vi "Read Parameter from Word.vi"(8 "error in":errorcluster, 9 "parameter definition":T1={"start index"=10, "size"=19, "encoding"=enum."BNR", "signed"=FALSE, "scale multiplier"=1.0, "scale offset"=0.0}, 11 "32-bit Word in":refnum<class "32-bit Word.lvclass">) -> (0 "error out":errorcluster, 2 "parameter value":dbl, 3 "32-bit Word out":refnum<class "32-bit Word.lvclass">)   [LabVIEW 2020, in "32-bit Word.lvclass"]
uses:
  32-bit Word.lvclass
  Parameter Definition.ctl
  Encoding and Decoding/Encoding.ctl
  32-bit Word.lvclass/32-bit Word.ctl
  696e3cb6-aa1b-4579-a134-6b36b9c1fdc9.vi
  8302f7cf-3c99-45e8-838e-289f83284f96.vi
  Read 32-Bit Word.vi
  696e3cb6-aa1b-4579-a134-6b36b9c1fdc9.vi/16a2565b-3c16-407b-a626-9da2a3da432e.vi
  8302f7cf-3c99-45e8-838e-289f83284f96.vi/0a001d06-2809-4638-8d0b-e017d2157007.vi
  Encoding and Decoding/BCD Decode Integer.vi
  Encoding and Decoding/BCD Decode Integer.vi/9a65bfc0-0d77-4ef3-ab58-63df1e1caa90.vi
  ARINC 429.lvclass
  Encoding and Decoding/Encoding and Decoding.lvlib
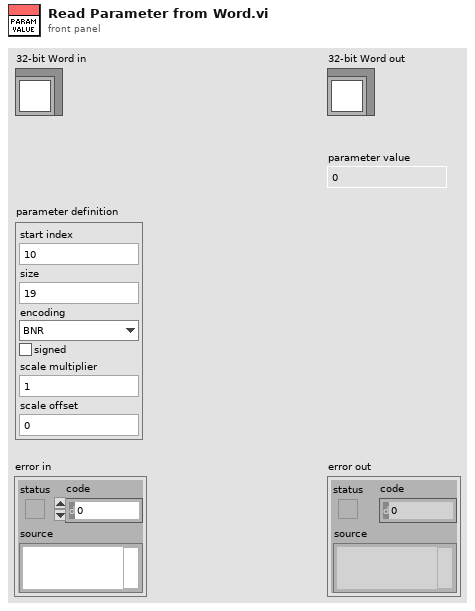
[diagram p1: front panel]
types:
  T1 = typedef "ARINC 429.lvclass/Parameter Definition.ctl" = cluster{"start index":i32, "size":i32, "encoding":T2, "signed":bool, "scale multiplier":dbl, "scale offset":dbl}
  T2 = typedef "Encoding and Decoding.lvlib/Encoding.ctl" = enum16{"BNR", "BCD", "Discrete"}
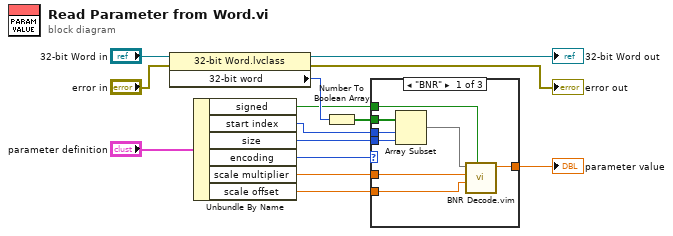
[diagram p0: block diagram]
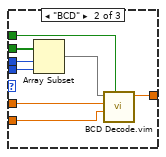
[diagram p2: hidden frame]
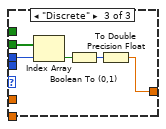
[diagram p3: hidden frame]
diagram:
  n1 = property on="Property Node" class="32-bit Word.lvclass"(reference="32-bit Word in", error in="error in") -> (reference out=→"32-bit Word out":refnum<class "32-bit Word.lvclass">, error out=→"error out":errorcluster, "32-bit word"=w10:u32)
  n2 = Unbundle By Name("parameter definition") -> ("signed"=w4:bool, "start index"=w2:i32, "size"=w1:i32, "encoding"=w14:T2, "scale multiplier"=w13:dbl, "scale offset"=w12:dbl)
  n3 = Number To Boolean Array(number=w10) -> (Boolean array=w3:bool[])
  n4 = case shown="\"BNR\"" w14 {
    tunnel: w13 -> [w22 w29 _]
    tunnel: w12 -> [w21 w28 _]
    tunnel: w4 -> [w20 w27 _]
    tunnel: [w19 w30 w31] -> w7
    tunnel: w3 -> [w18 w26 w35]
    tunnel: w2 -> [w17 w25 w34]
    tunnel: w1 -> [w16 w24 _]
    frame "BNR" {
      n5 = Array Subset(array=w18, index=w17, length=w16) -> (w15:bool[])
      n6 = call "BNR Decode.vim"("signed"=w20, "scale offset"=w21, "scale multiplier"=w22, "BNR encoded value"=w15) -> ("value"=w19:dbl)  [unwired: 7 in]
    }
    frame "BCD" {
      n7 = Array Subset(array=w26, index=w25, length=w24) -> (w23:bool[])
      n8 = call "BCD Decode.vim"("signed"=w27, "scale offset"=w28, "scale multiplier"=w29, "BCD encoded value"=w23) -> ("value"=w30:dbl)  [unwired: 7 in]
    }
    frame "Discrete" {
      n9 = Index Array(array=w35, index=w34) -> (element=w33:bool)
      n10 = Boolean To (0,1)(Boolean=w33) -> (0, 1=w32:i16)
      n11 = To Double Precision Float(number=w32) -> (double precision float=w31:dbl)
    }
  }
  "parameter value" <- w7
